vi "sCMOS_init_merFISH.vi"(3 "error in":errorcluster, 4 "Start acquisition":bool, 5 "handle":u32) -> (0 "error out":errorcluster {"code" format="%.0x"})   [LabVIEW 2015]
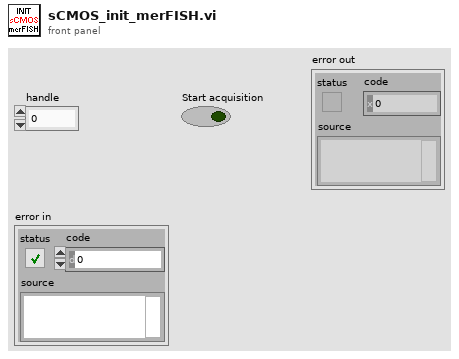
[diagram p1: front panel]
types:
  T1 = cluster{"Mode":u32, "Polarity":u32, "Times":u32, "Delay":dbl}
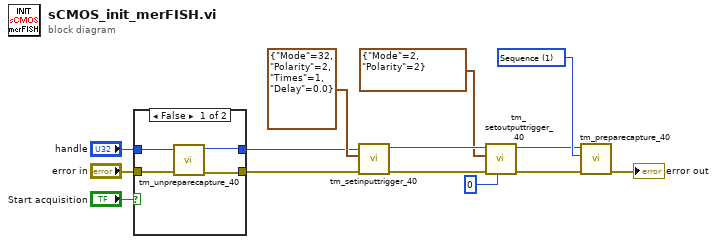
[diagram p0: block diagram]
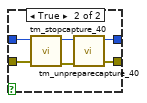
[diagram p2: hidden frame]
diagram:
  w14 = 1 items=["Snap", "Sequence"] ("Capture mode")
  n1 = case shown="False" "Start acquisition" {
    tunnel: "error in" -> [w16 w24]
    tunnel: [w15 w20] -> w1
    tunnel: "handle" -> [w18 w23]
    tunnel: [w17 w19] -> w2
    frame False {
      n2 = call <userlib>:"tm_unpreparecapture_40.vi"("error in (no error)"=w16, "Handle in"=w18) -> ("error out"=w15:errorcluster, "Handle out"=w17:u32)  [unwired: 8 in]
    }
    frame True {
      n3 = call <userlib>:"tm_stopcapture_40.vi"("error in (no error)"=w24, "Handle in"=w23) -> ("error out"=w22:errorcluster, "Handle out"=w21:u32)  [unwired: 8 in]
      n4 = call <userlib>:"tm_unpreparecapture_40.vi"("error in (no error)"=w22, "Handle in"=w21) -> ("error out"=w20:errorcluster, "Handle out"=w19:u32)  [unwired: 8 in]
    }
  }
  n5 = call <userlib>:"tm_setinputtrigger_40.vi"("error in (no error)"=w1, "Parameters"=T1 {"Mode"=32, "Polarity"=2, "Times"=1, "Delay"=0.0}, "Handle in"=w2) -> ("error out"=w10:errorcluster, "Handle out"=w8:u32)  [unwired: 7 in]
  n6 = call <userlib>:"tm_setoutputtrigger_40.vi"("Port"=0, "error in (no error)"=w10, "Type"=cluster{"Mode":u32, "Polarity":u32} {"Mode"=2, "Polarity"=2}, "Handle in"=w8) -> ("error out"=w9:errorcluster, "Handle out"=w7:u32)  [unwired: 6 in]
  n7 = call <userlib>:"tm_preparecapture_40.vi"("error in (no error)"=w9, "Capture mode"=w14, "Handle in"=w7) -> ("error out"=→"error out":errorcluster)  [unwired: 5 in, 3 out]
